vi "SRV_Calculate Window Size Bounds.vi"(5 "FP Window Bounds":T1, 9 "FP Width-Height":cluster{"Width":i16, "Height":i16}) -> (6 "FP Window Bounds out":T1)   [LabVIEW 2014]
uses:
  <vilib>/Utility/miscctls.llb/LVRectTypeDef.ctl
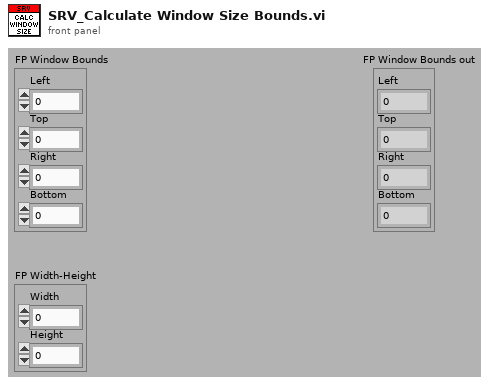
[diagram p1: front panel]
types:
  T1 = typedef "LVRectTypeDef.ctl" = cluster{"Left":i16, "Top":i16, "Right":i16, "Bottom":i16}
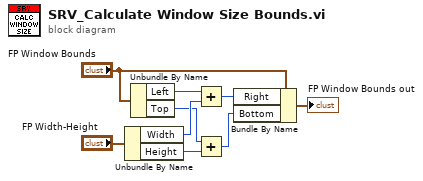
[diagram p0: block diagram]
diagram:
  n1 = Unbundle By Name("FP Width-Height") -> ("Width"=w5:i16, "Height"=w1:i16)
  n2 = Unbundle By Name("FP Window Bounds") -> ("Left"=w6:i16, "Top"=w2:i16)
  n3 = Add(x=w6, y=w5) -> (x+y=w4:i16)
  n4 = Add(x=w2, y=w1) -> (x+y=w3:i16)
  n5 = Bundle By Name(cluster="FP Window Bounds", "Right"=w4, "Bottom"=w3) -> (→"FP Window Bounds out":T1)
